vi "CloseSession.vi"(8 "error in (no error)":errorcluster, 10 "gRPCid":T4, 11 "ctet_smu":T1) -> (0 "error out":errorcluster, 3 "ctet_smu out":T1)   [LabVIEW 2019, in "ctet_smu User Library.lvlib"]
uses:
  ctet_smu User Library.lvlib
  Servers/ctet_smu/gRPC lvSupport/Server API/typeDefs/grpcId.ctl
  Types/ctet_smu.ctl
  Servers/ctet_smu/ctet_smu Class/RPC Messages/measurementservice_SMUConfigResponse/measurementservice_SMUConfigResponse_Data.ctl
  Servers/ctet_smu/ctet_smu Class/RPC Messages/measurementservice_ErrorOut/measurementservice_ErrorOut_Data.ctl
  Servers/ctet_smu/ctet_smu Class/RPC Messages/measurementservice_SMUCloseSessionResponse/measurementservice_SMUCloseSessionResponse_Data.ctl
  Servers/ctet_smu/ctet_smu Class/ctet_smu.lvclass
  Servers/ctet_smu/gRPC lvSupport/gprc-lvsupport.lvlib
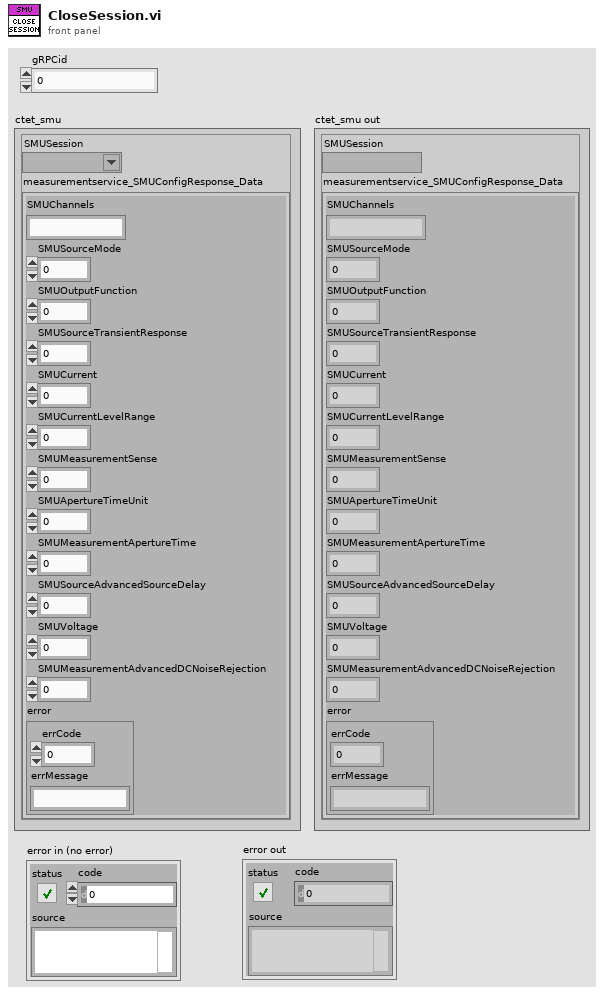
[diagram p1: front panel]
types:
  T1 = typedef "ctet_smu User Library.lvlib/ctet_smu.ctl" = cluster{"SMUSession":refnum<k15>, "measurementservice_SMUConfigResponse_Data":T2}
  T2 = typedef "ctet_smu.lvlib/ctet_smu.lvclass/measurementservice_SMUConfigResponse_Data.ctl" = cluster{"SMUChannels":string, "SMUSourceMode":i64, "SMUOutputFunction":i64, "SMUSourceTransientResponse":i64, "SMUCurrent":dbl, "SMUCurrentLevelRange":dbl, "SMUMeasurementSense":i64, "SMUApertureTimeUnit":i64, "SMUMeasurementApertureTime":dbl, "SMUSourceAdvancedSourceDelay":dbl, "SMUVoltage":dbl, "SMUMeasurementAdvancedDCNoiseRejection":i64, "error":T3}
  T3 = typedef "ctet_smu.lvlib/ctet_smu.lvclass/measurementservice_ErrorOut_Data.ctl" = cluster{"errCode":i64, "errMessage":string}
  T4 = typedef "ctet_smu.lvlib/gprc-lvsupport.lvlib/grpcId.ctl" = u64
  T5 = typedef "ctet_smu.lvlib/ctet_smu.lvclass/measurementservice_SMUCloseSessionResponse_Data.ctl" = cluster{"error":T3}
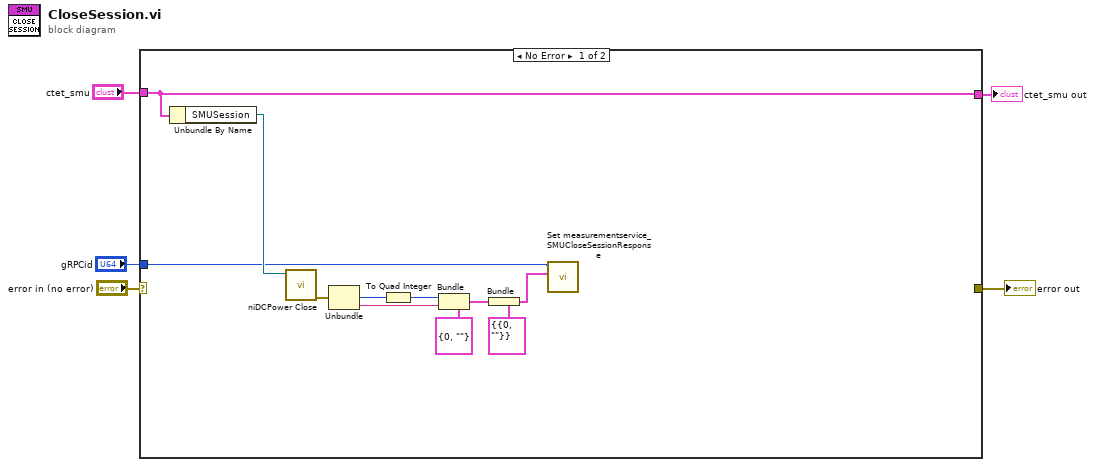
[diagram p0: block diagram]
diagram:
  n1 = case shown="No Error" "error in (no error)" {
    selector: "error in (no error)" -> [_ w18]
    tunnel: [_ w18] -> w5
    tunnel: "gRPCid" -> [w10 _]
    tunnel: "ctet_smu" -> [w11 w17]
    tunnel: [w11 w17] -> w1
    frame No Error {
      n2 = Unbundle By Name(w11) -> ("SMUSession"=w12:refnum<k15>)
      n3 = call <instrlib>:"niDCPower Close.vi"("instrument handle"=w12) -> ("error out"=w16:errorcluster)  [unwired: 10 in]
      n4 = Unbundle(w16) -> ("code"=w14:i32, "source"=w15:string)  [unwired: 1 out]
      n5 = To Quad Integer(1:w14) -> (0:w13:i64)
      n6 = Bundle(cluster=T3 {"errCode"=0, "errMessage"=""} ("error"), "errCode"=w13, "errMessage"=w15) -> (w6:T3)
      n7 = Bundle(cluster=T5 {"error"={"errCode"=0, "errMessage"=""}} ("Message Data"), "error"=w6) -> (w8:T5)
      n8 = call "Set measurementservice_SMUCloseSessionResponse.vi"("Message Data"=w8, "gRPCid"=w10) -> ()  [unwired: 9 in, 1 out]
    }
    frame Error {
    }
  }
  "error out" <- w5
  "ctet_smu out" <- w1
